vi "Read Marker Values[].vi"(9 "ColorScale in":refnum<class "ColorScale.lvclass">) -> (3 "ColorScale out":refnum<class "ColorScale.lvclass">, 4 "Marker Values[]":cluster{dbl, u32}[](array[cluster]))   [LabVIEW 2014, in "ColorScale.lvclass"]
uses:
  ColorScale.lvclass
  ColorScale.lvclass/ColorScale.ctl
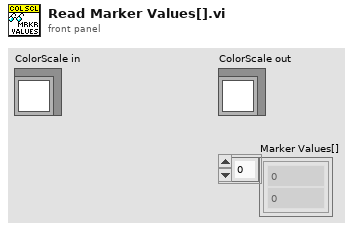
[diagram p1: front panel]
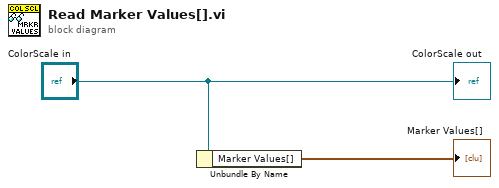
[diagram p0: block diagram]
diagram:
  n1 = Unbundle By Name("ColorScale in") -> ("Marker Values[]"=→"Marker Values[]":cluster{dbl, u32}[])
  "ColorScale out" <- "ColorScale in"
